vi "MotionProfileGenerator.vi"(1 "Starting Position (rotations)":dbl, 2 "Travel Distance (rotations)":dbl, 3 "Acceleration Ramp Time (ms)":dbl=1.0 min=1.0, 4 "Velocity Ramp Time (ms)":dbl min=1.0, 5 "Trajectory Point Interval (ms)":i32=1 min=1, 6 "Maximum Travel Speed (rpm)":dbl min=0.0) -> (0 "Trajectory Points":T1[](array[typedef]))   [LabVIEW 2017]
uses:
  Type.Def/TrajectoryPoint.ctl
panel:
  out "Input":bool
  out "T4":dbl
  out "fl2":dbl
  out "fl1":dbl
  out "n":dbl
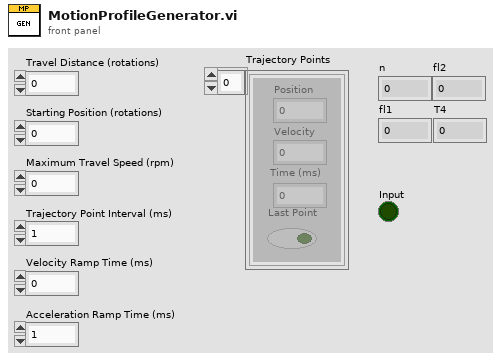
[diagram p1: front panel]
types:
  T1 = typedef "TrajectoryPoint.ctl" = cluster{"Position ":dbl, "Velocity ":dbl, "Time (ms)":i32, "Last Point":bool}
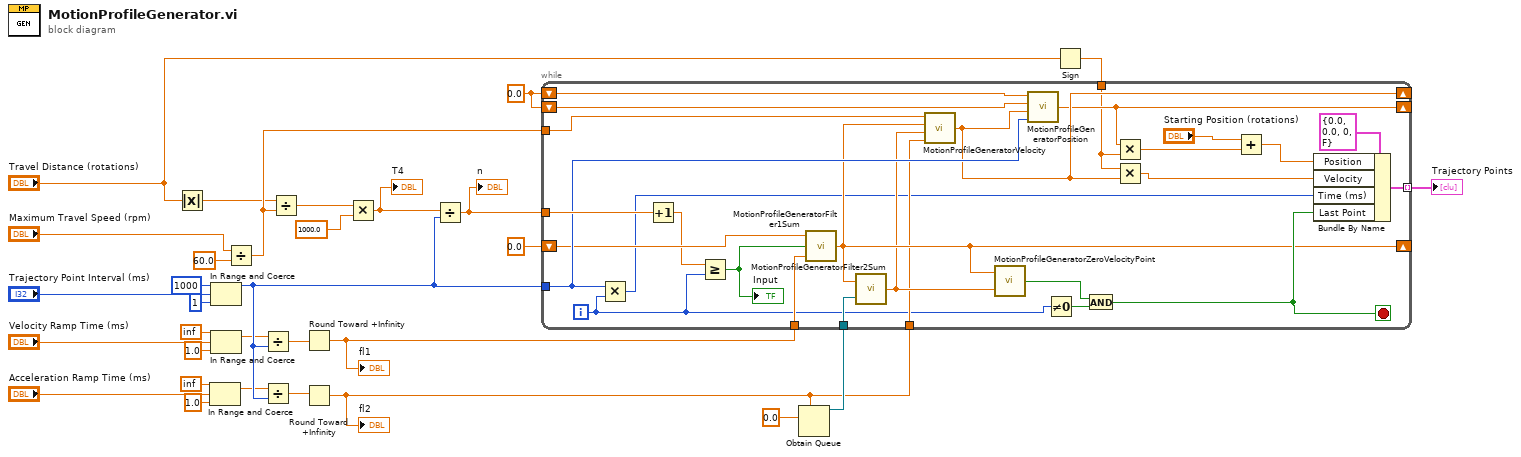
[diagram p0: block diagram]
diagram:
  w4 = 0.0
  n1 = Absolute Value(x="Travel Distance (rotations)") -> (abs(x)=w18:dbl)
  n2 = In Range and Coerce(upper limit=inf, x="Acceleration Ramp Time (ms)", lower limit=1.0) -> (coerced(x)=w11:dbl)  [unwired: 1 out]
  n3 = In Range and Coerce(upper limit=1000, x="Trajectory Point Interval (ms)", lower limit=1) -> (coerced(x)=w15:i32)  [unwired: 1 out]
  n4 = In Range and Coerce(upper limit=inf, x="Velocity Ramp Time (ms)", lower limit=1.0) -> (coerced(x)=w12:dbl)  [unwired: 1 out]
  n5 = Divide(x="Maximum Travel Speed (rpm)", y=60.0) -> (x/y=w19:dbl)
  n6 = Divide(x=w12, y=w15) -> (x/y=w26:dbl)
  n7 = Divide(x=w11, y=w15) -> (x/y=w27:dbl)
  n8 = Divide(x=w18, y=w19) -> (x/y=w29:dbl)
  n9 = Round Toward +Infinity(x=w26) -> (ceil(x): smallest int >= x=w17:dbl)
  "fl1" <- w17
  n10 = Round Toward +Infinity(x=w27) -> (ceil(x): smallest int >= x=w16:dbl)
  "fl2" <- w16
  n11 = Multiply(x=w29, y=1000.0) -> (x*y=w25:dbl)
  "T4" <- w25
  n12 = Divide(x=w25, y=w15) -> (x/y=w24:dbl)
  "n" <- w24
  n13 = Obtain Queue(max queue size (-1, unlimited)=w16, element data type=0.0) -> (queue out=w21:refnum<queue>)  [unwired: 3 in, 2 out]
  n14 = Sign(1:"Travel Distance (rotations)") -> (0:w2:dbl)
  n15 = while {
    tunnel: w15 -> [w52]
    tunnel: w24 -> [w58]
    shift-right: [w46] -> _
    shift-left: 0.0 -> [w48]
    tunnel: w21 -> [w50]
    tunnel: [w55] -> w20 mode=indexing
    tunnel: w16 -> [w44]
    tunnel: w19 -> [w47]
    shift-right: [w39] -> _
    shift-left: w4 -> [w53]
    shift-right: [w36] -> _
    shift-left: w4 -> [w43]
    tunnel: w17 -> [w49]
    tunnel: w2 -> [w35]
    i -> [w42]
    stop <- w54 stop-if-true
    n16 = Multiply(x=w52, y=w42) -> (x*y=w32:i32)
    n17 = Increment(x=w58) -> (x+1=w41:dbl)
    n18 = Greater Or Equal?(x=w41, y=w42) -> (x >= y?=w40:bool)
    "Input" <- w40
    n19 = call "MotionProfileGeneratorFilter1Sum.vi"("fl1"=w49, "Input"=w40, "Previous Filter1Sum"=w48) -> ("Filter1Sum"=w46:dbl)
    n20 = call "MotionProfileGeneratorFilter2Sum.vi"("Filter Queue"=w50, "Filter1Sum"=w46) -> ("Filter2Sum"=w45:dbl)
    n21 = call "MotionProfileGeneratorVelocity.vi"("FL2"=w44, "filter2sum"=w45, "Filter1Sum"=w46, "Maximum Travel Speed (rps)"=w47) -> ("Velocity"=w39:dbl)
    n22 = call "MotionProfileGeneratorZeroVelocityPoint.vi"("Filter2Sum"=w45, "Filter1Sum"=w46) -> ("Zero Velocity"=w51:bool)
    n23 = call "MotionProfileGeneratorPosition.vi"("Trajectory Point Interval (ms)"=w52, "Velocity"=w39, "Previous Position"=w43, "Previous Velocity"=w53) -> ("Position"=w36:dbl)
    n24 = Not Equal To 0?(x=w42) -> (x != 0?=w57:bool)
    n25 = And(x=w51, y=w57) -> (x .and. y?=w54:bool)
    n26 = Multiply(x=w36, y=w35) -> (x*y=w34:dbl)
    n27 = Multiply(x=w35, y=w39) -> (x*y=w37:dbl)
    n28 = Add(x="Starting Position (rotations)", y=w34) -> (x+y=w33:dbl)
    n29 = Bundle By Name(cluster=T1 {"Position "=0.0, "Velocity "=0.0, "Time (ms)"=0, "Last Point"=FALSE} ("trajectory point"), "Position"=w33, "Velocity"=w37, "Time (ms)"=w32, "Last Point"=w54) -> (w55:T1)
  }
  "Trajectory Points" <- w20
